vi "Fall_in_Air.vi"() -> ()   [LabVIEW 2022 SP3]
panel:
  out "Terminal Velocity\nfrom Data (m/s)":string
  out "Calculated Terminal \nVelocity (m/s)":dbl
  out "Cross Sectional Area (m**2)":dbl
  out "b":dbl
  out "Velocity v. Time":cluster{dbl, dbl}[](graph)
  in  "Number of Samples":dbl
  in  "dt":dbl
  in  "Mass (kg)":dbl
  in  "Gravitational Acceleration (m/s**2)":dbl
  in  "V0 (m/s)":dbl
  in  "Air Density (kg/m**3)":dbl
  in  "Radius (m)":dbl
  in  "Drag Coefficient":dbl
  # "Resultant Values:"
  # "Object Parameters:"
  # "Environment:"
  # "Timing:"
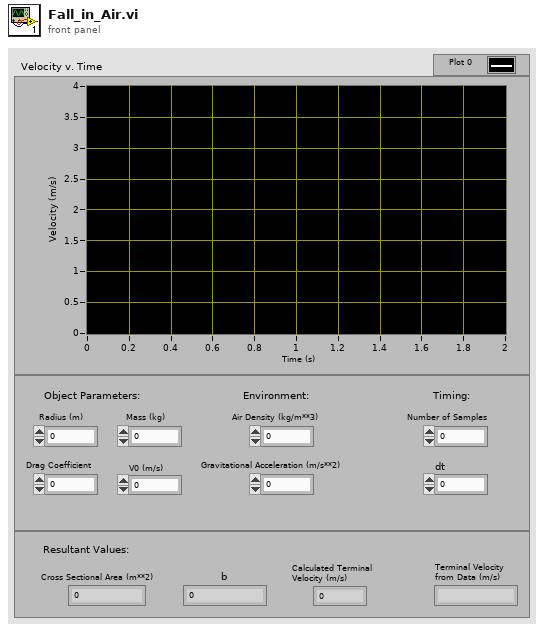
[diagram p1: front panel]
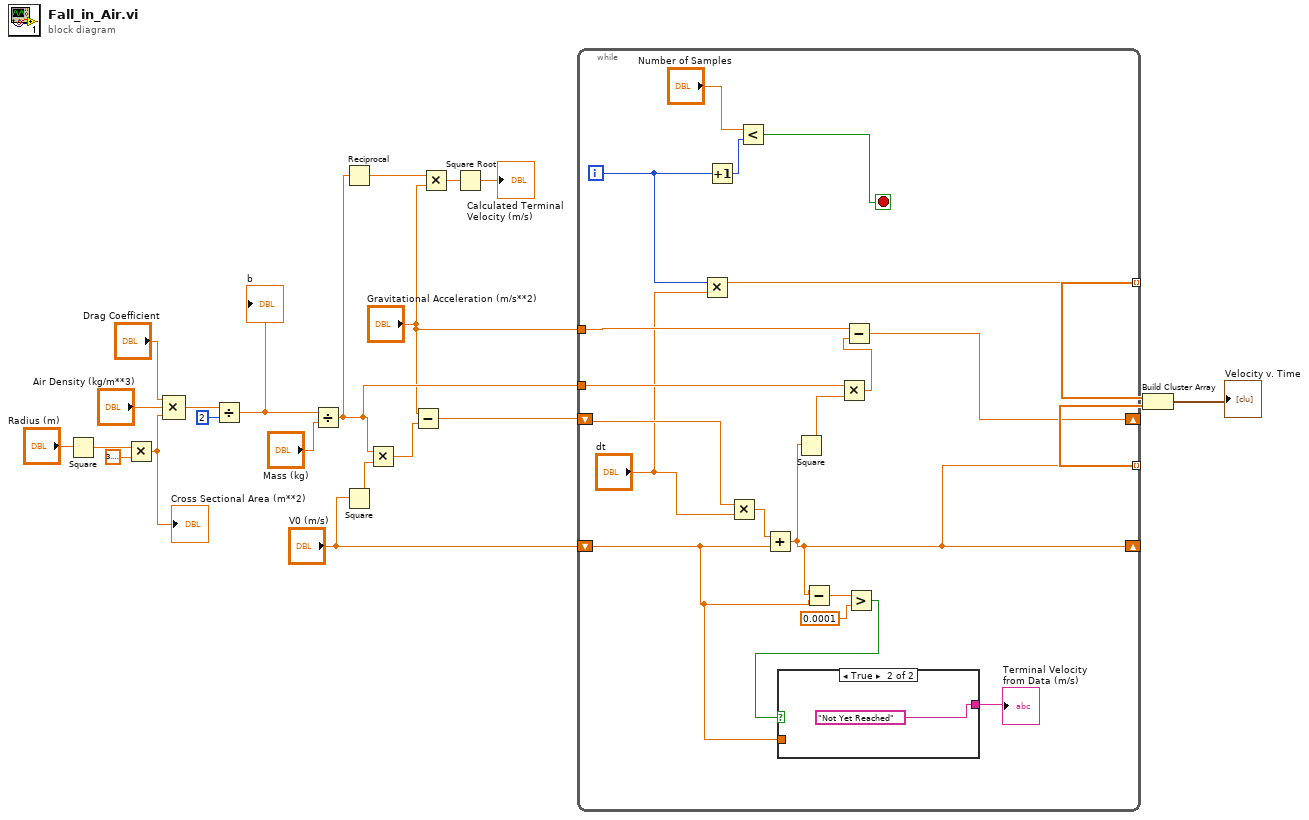
[diagram p0: block diagram]
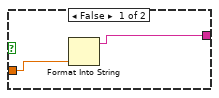
[diagram p2: hidden frame]
diagram:
  n1 = Square(x="Radius (m)") -> (x^2=w18:dbl)
  n2 = Multiply(x=w18, y=3.141592653589793) -> (x*y=w21:dbl)
  "Cross Sectional Area (m**2)" <- w21
  n3 = Compound Arithmetic op=MULTIPLY("Drag Coefficient", "Air Density (kg/m**3)", w21) -> (w22:dbl)
  n4 = Divide(x=w22, y=2) -> (x/y=w13:dbl)
  "b" <- w13
  n5 = Divide(x=w13, y="Mass (kg)") -> (x/y=w5:dbl)
  n6 = Reciprocal(x=w5) -> (1/x=w4:dbl)
  n7 = Square(x="V0 (m/s)") -> (x^2=w11:dbl)
  n8 = Multiply(x=w5, y=w11) -> (x*y=w10:dbl)
  n9 = Subtract(x="Gravitational Acceleration (m/s**2)", y=w10) -> (x-y=w9:dbl)
  n10 = Multiply(x=w4, y="Gravitational Acceleration (m/s**2)") -> (x*y=w2:dbl)
  n11 = Square Root(x=w2) -> (sqrt(x)=→"Calculated Terminal \nVelocity (m/s)":dbl)
  n12 = while {
    shift-right: [w33] -> _
    shift-left: w9 -> [w38]
    shift-right: [w27] -> _
    shift-left: "V0 (m/s)" -> [w24]
    tunnel: w5 -> [w37]
    tunnel: "Gravitational Acceleration (m/s**2)" -> [w34]
    tunnel: [w27] -> w8 mode=indexing
    tunnel: [w30] -> w7 mode=indexing
    i -> [w31]
    stop <- w41 stop-if-true
    n13 = Multiply(x=w31, y="dt") -> (x*y=w30:dbl)
    n14 = Increment(x=w31) -> (x+1=w40:i32)
    n15 = Multiply(x=w38, y="dt") -> (x*y=w39:dbl)
    n16 = Less?(x="Number of Samples", y=w40) -> (x < y?=w41:bool)
    n17 = Add(x=w39, y=w24) -> (x+y=w27:dbl)
    n18 = Square(x=w27) -> (x^2=w36:dbl)
    n19 = Subtract(x=w27, y=w24) -> (x-y=w28:dbl)
    n20 = Multiply(x=w37, y=w36) -> (x*y=w35:dbl)
    n21 = Subtract(x=w34, y=w35) -> (x-y=w33:dbl)
    n22 = Greater?(x=w28, y=0.0001) -> (0:w25:bool)
    n23 = case shown="True" w25 {
      tunnel: [w42 "Not Yet Reached"] -> w23
      tunnel: w24 -> [w43 _]
      frame False {
        n24 = Format Into String(w43) -> (resulting string=w42:string)  [unwired: 3 in, 1 out]
      }
      frame True {
      }
    }
    "Terminal Velocity\nfrom Data (m/s)" <- w23
  }
  n25 = Build Cluster Array(w7, w8) -> (→"Velocity v. Time":cluster{dbl, dbl}[])
